vi "Change Password.vi"(8 "error in (no error)":errorcluster, 9 "Salt":string, 10 "New Password":string, 11 "Content in":T1) -> (0 "error out":errorcluster, 3 "Content out":T1)   [LabVIEW 2018, in "VI-Hacker.lvlib"]
uses:
  VI-Hacker.lvlib
  <vilib>/ErrorRing/Error Ring.xnode
  <vilib>/Utility/error.llb/Error Cluster From Error Code.vi
  TypeDefs/Block.ctl
  TypeDefs/Content.ctl
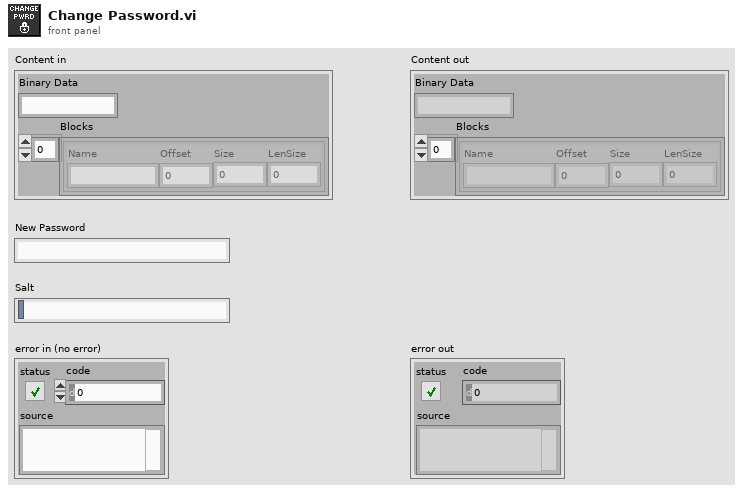
[diagram p1: front panel]
types:
  T1 = typedef "VI-Hacker.lvlib/Content.ctl" = cluster{"Binary Data":string, "Blocks":T2[]}
  T2 = typedef "VI-Hacker.lvlib/Block.ctl" = cluster{"Name":string, "Offset":i32, "Size":i32, "LenSize":i32}
  T3 = typedef "VI-Hacker.lvlib/Block vers.ctl" = cluster{"Version":cluster{"Major":u8, "Minor":u8, "Fix":u8, "Build":u8}, "Stage":enum8{"Development", "Alpha", "Beta", "Release"}, "Flags":u16, "VersionString":string, "VersionInfo":string}
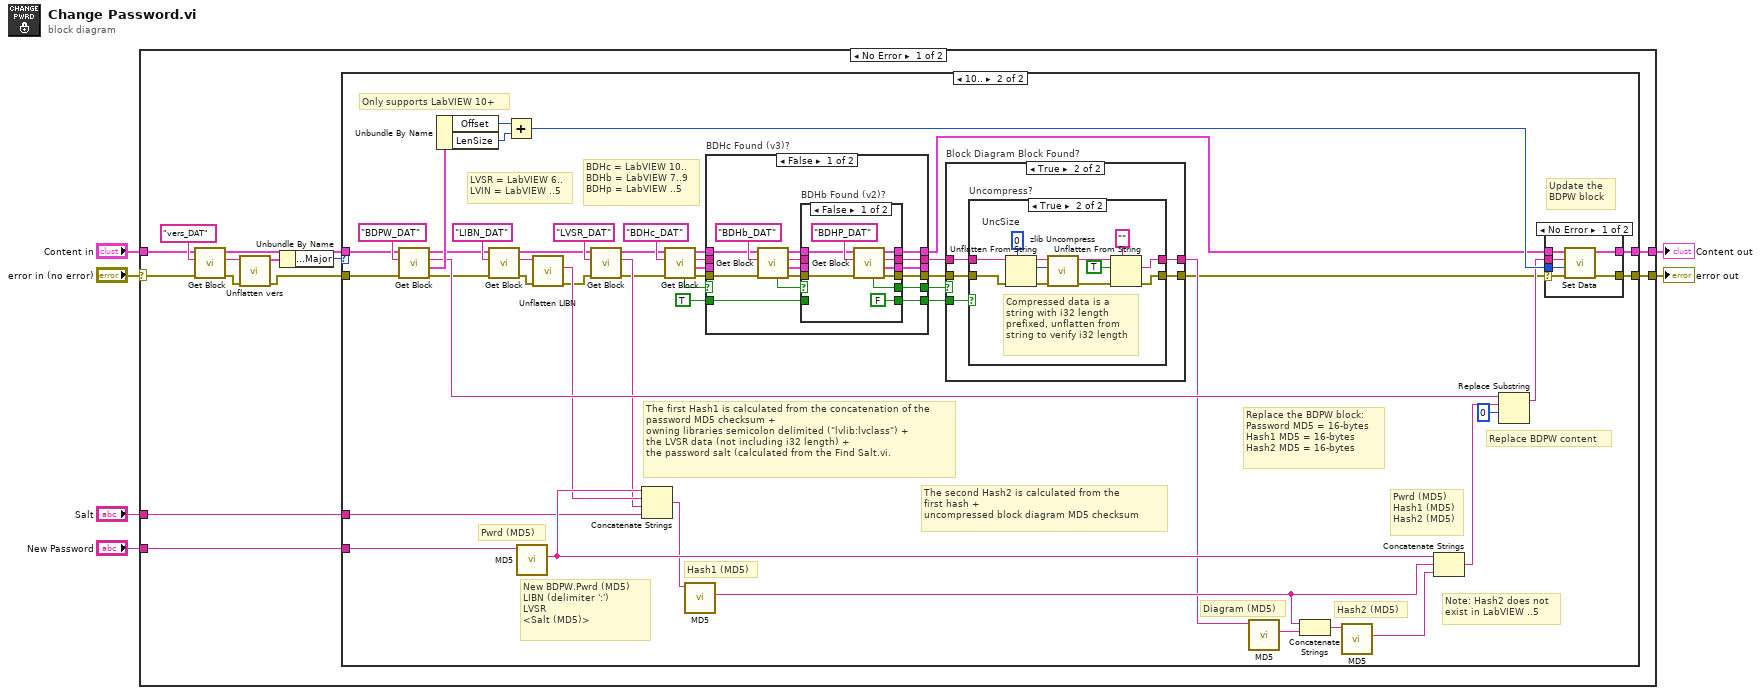
[diagram p0: block diagram]
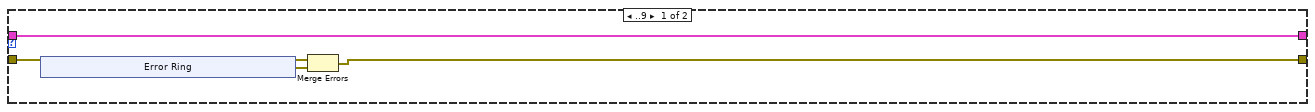
[diagram p2: hidden frame]
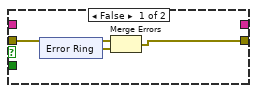
[diagram p4: hidden frame]
diagram:
  n1 = case shown="No Error" "error in (no error)" {
    selector: "error in (no error)" -> [w11 w146]
    tunnel: "Content in" -> [w8 w145]
    tunnel: "New Password" -> [w19 _]
    tunnel: [w18 w146] -> w3
    tunnel: [w17 w145] -> w2
    tunnel: "Salt" -> [w16 _]
    frame No Error {
      n2 = call "Get Block.vi"("error in (no error)"=w11, "Block Name"="vers_DAT", "Content in"=w8) -> ("error out"=w14:errorcluster, "Data out"=w13:string, "Content out"=w9:T1)  [unwired: 4 in, 2 out]
      n3 = call "Unflatten vers.vi"("error in (no error)"=w14, "Data in"=w13) -> ("error out"=w10:errorcluster, "vers"=w12:T3)  [unwired: 8 in]
      n4 = Unbundle By Name(w12) -> ("Version.Major"=w7:u8)
      n5 = case shown="10.." w7 {
        tunnel: w19 -> [_ w72]
        tunnel: [w21 w70] -> w18
        tunnel: [w22 w69] -> w17
        tunnel: w16 -> [_ w51]
        tunnel: w10 -> [w23 w46]
        tunnel: w9 -> [w22 w45]
        frame ..9 {
          n6 = xnode "Error Ring"() -> ("error out"=w20:errorcluster)
          n7 = Merge Errors(w23, w20) -> (w21:errorcluster)
        }
        frame 10.. {
          # "Update the\nBDPW block"
          # "Replace BDPW content"
          # "Note: Hash2 does not\nexist in LabVIEW ..5"
          # "Replace the BDPW block:\nPassword MD5 = 16-bytes\nHash1 MD5 = 16-bytes\nHash2 MD5 = 16-bytes"
          # "The second Hash2 is calculated from the\nfirst hash +\nuncompressed block diagram MD5 checksum"
          # "The first Hash1 is calculated from the concatenation of the\npassword MD5 checksum +\nowning libraries semicolon delimited (\"lvlib:lvclass\") +\nthe LVSR data (not including i32 length) +\nthe password salt (calculated from the Find Salt.vi."
          # "LVSR = LabVIEW 6..\nLVIN = LabVIEW ..5"
          # "BDHc = LabVIEW 10..\nBDHb = LabVIEW 7..9\nBDHp = LabVIEW ..5"
          # "Diagram (MD5)"
          # "Hash2 (MD5)"
          # "Hash1 (MD5)"
          # "Pwrd (MD5)"
          # "New BDPW.Pwrd (MD5)\nLIBN (delimiter ':')\nLVSR\n<Salt (MD5)>"
          # "Only supports LabVIEW 10+"
          # "Pwrd (MD5)\nHash1 (MD5)\nHash2 (MD5)"
          n8 = call "Get Block.vi"("error in (no error)"=w46, "Block Name"="BDPW_DAT", "Content in"=w45) -> ("error out"=w60:errorcluster, "Block out"=w73:T2, "Data out"=w71:string, "Content out"=w61:T1)  [unwired: 4 in, 1 out]
          n9 = Unbundle By Name(w73) -> ("Offset"=w68:i32, "LenSize"=w67:i32)
          n10 = call "Get Block.vi"("error in (no error)"=w60, "Block Name"="LIBN_DAT", "Content in"=w61) -> ("error out"=w58:errorcluster, "Data out"=w59:string, "Content out"=w53:T1)  [unwired: 4 in, 2 out]
          n11 = Add(x=w68, y=w67) -> (x+y=w66:i32)
          n12 = call "MD5.vi"("Message String"=w72) -> ("MD5 (16-bytes)"=w57:string)  [unwired: 9 in, 1 out]
          n13 = call "Unflatten LIBN.vi"("error in (no error)"=w58, "Data in"=w59) -> ("error out"=w54:errorcluster, "Libraries (MD5 Salt)"=w56:string)  [unwired: 7 in, 1 out]
          n14 = call "Get Block.vi"("error in (no error)"=w54, "Block Name"="LVSR_DAT", "Content in"=w53) -> ("error out"=w48:errorcluster, "Data out"=w52:string, "Content out"=w49:T1)  [unwired: 4 in, 2 out]
          n15 = Concatenate Strings(w57, w56, w52, w51) -> (w47:string)
          n16 = call "Get Block.vi"("error in (no error)"=w48, "Block Name"="BDHc_DAT", "Content in"=w49) -> ("error out"=w39:errorcluster, "Block out"=w36:T2, "Data out"=w37:string, "Content out"=w40:T1, "Found?"=w38:bool)  [unwired: 4 in]
          n17 = call "MD5.vi"("Message String"=w47) -> ("MD5 (16-bytes)"=w44:string)  [unwired: 9 in, 1 out]
          n18 = case "BDHc Found (v3)?" shown="False" w38 {
            selector: w38 -> [_ w140]
            tunnel: w40 -> [w122 w144]
            tunnel: w39 -> [w121 w143]
            tunnel: [w118 w143] -> w35
            tunnel: [w115 w144] -> w28
            tunnel: w37 -> [_ w142]
            tunnel: w36 -> [_ w141]
            tunnel: [w116 w142] -> w34
            tunnel: [w117 w141] -> _
            tunnel: [w110 w140] -> w31
            tunnel: [w109 w139] -> w33
            tunnel: TRUE -> [w114 w139]
            frame False {
              n19 = call "Get Block.vi"("error in (no error)"=w121, "Block Name"="BDHb_DAT", "Content in"=w122) -> ("error out"=w119:errorcluster, "Block out"=w111:T2, "Data out"=w112:string, "Content out"=w120:T1, "Found?"=w113:bool)  [unwired: 4 in]
              n20 = case "BDHb Found (v2)?" shown="False" w113 {
                selector: w113 -> [_ w133]
                tunnel: w120 -> [w131 w137]
                tunnel: w119 -> [w130 w138]
                tunnel: [w129 w138] -> w118
                tunnel: [w128 w135] -> w117
                tunnel: [w127 w136] -> w116
                tunnel: [w126 w137] -> w115
                tunnel: w114 -> [_ w134]
                tunnel: w112 -> [_ w136]
                tunnel: w111 -> [_ w135]
                tunnel: [w125 w133] -> w110
                tunnel: [FALSE w134] -> w109
                frame False {
                  n21 = call "Get Block.vi"("error in (no error)"=w130, "Block Name"="BDHP_DAT", "Content in"=w131) -> ("error out"=w129:errorcluster, "Block out"=w128:T2, "Data out"=w127:string, "Content out"=w126:T1, "Found?"=w125:bool)  [unwired: 4 in]
                }
                frame True {
                }
              }
            }
            frame True {
            }
          }
          n22 = case "Block Diagram Block Found?" shown="True" w31 {
            tunnel: w35 -> [w85 w94]
            tunnel: w34 -> [_ w93]
            tunnel: w33 -> [_ w92]
            tunnel: [w84 w91] -> w29
            tunnel: [_ w90] -> w30
            frame False {
              n23 = xnode "Error Ring"() -> ("error out"=w83:errorcluster)
              n24 = Merge Errors(w85, w83) -> (w84:errorcluster)
            }
            frame True {
              n25 = case "Uncompress?" shown="True" w92 {
                tunnel: w94 -> [w95 w108]
                tunnel: w93 -> [w96 w103]
                tunnel: [w95 w101] -> w91
                tunnel: [w96 w97] -> w90
                frame False {
                }
                frame True {
                  w106 = u32 0  # UncSize
                  # "Compressed data is a\nstring with i32 length\nprefixed, unflatten from\nstring to verify i32 length"
                  n26 = Unflatten From String(type=w106, binary string=w103, error in (no error)=w108) -> (rest of the binary string=w104:string, value=w105:u32, error out=w107:errorcluster)  [unwired: 2 in]
                  n27 = call "zlib Uncompress.vi"("error in (no error)"=w107, "Uncompressed Size in"=w105, "Compressed Data in"=w104) -> ("error out"=w102:errorcluster, "Uncompressed Data out"=w100:string)  [unwired: 6 in, 1 out]
                  n28 = Unflatten From String(type="", binary string=w100, data includes array or string size? (T)=TRUE, error in (no error)=w102) -> (value=w97:string, error out=w101:errorcluster)  [unwired: 1 in, 1 out]
                }
              }
            }
          }
          n29 = call "MD5.vi"("Message String"=w30) -> ("MD5 (16-bytes)"=w43:string)  [unwired: 9 in, 1 out]
          n30 = Concatenate Strings(w44, w43) -> (w42:string)
          n31 = call "MD5.vi"("Message String"=w42) -> ("MD5 (16-bytes)"=w41:string)  [unwired: 9 in, 1 out]
          n32 = Concatenate Strings(w57, w44, w41) -> (w64:string)
          n33 = Replace Substring(3:0 ("offset (0)"), 4:w64, 5:w71) -> (1:w65:string)  [unwired: 1 in, 1 out]
          n34 = case shown="No Error" w29 {
            selector: w29 -> [w76 w82]
            tunnel: [w80 w82] -> w70
            tunnel: [w79 w81] -> w69
            tunnel: w66 -> [w78 _]
            tunnel: w65 -> [w77 _]
            tunnel: w28 -> [w75 w81]
            frame No Error {
              n35 = call "Set Data.vi"("error in (no error)"=w76, "Offset"=w78, "Data in"=w77, "Content in"=w75) -> ("error out"=w80:errorcluster, "Content out"=w79:T1)  [unwired: 6 in]
            }
            frame Error {
            }
          }
        }
      }
    }
    frame Error {
    }
  }
  "error out" <- w3
  "Content out" <- w2
